vi "RPNSolver.vi"(7 "error in":errorcluster, 9 "Variable Value Array":sgl[](array[numeric]), 10 "Parsed Expression In":T1) -> (0 "error out":errorcluster, 2 "Numeric":sgl format="%#_18f", 3 "Parsed Expression Out":T1)   [LabVIEW 2014, in "MathLoop.lvlib"]
doc: "Resuelve las operaciones matemáticas."
uses:
  MathLoop.lvlib
  TypeDefs/ParsedExpression.ctl
  TypeDefs/typeMed.ctl
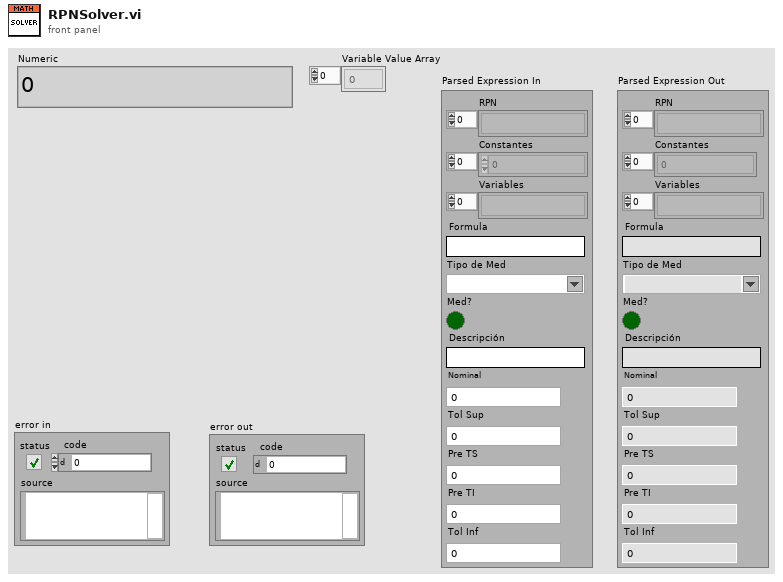
[diagram p1: front panel]
types:
  T1 = typedef "MathLoop.lvlib/ParsedExpression.ctl" = cluster{"RPN ":string[], "Constantes":sgl[], "Variables":string[], "Formula":string, "Tipo de Med":T2, "Med?":bool, "Descripción":string, "Nominal":sgl, "Tol Sup":sgl, "Pre TS":sgl, "Pre TI":sgl, "Tol Inf":sgl}
  T2 = typedef "MathLoop.lvlib/typeMed.ctl" = string
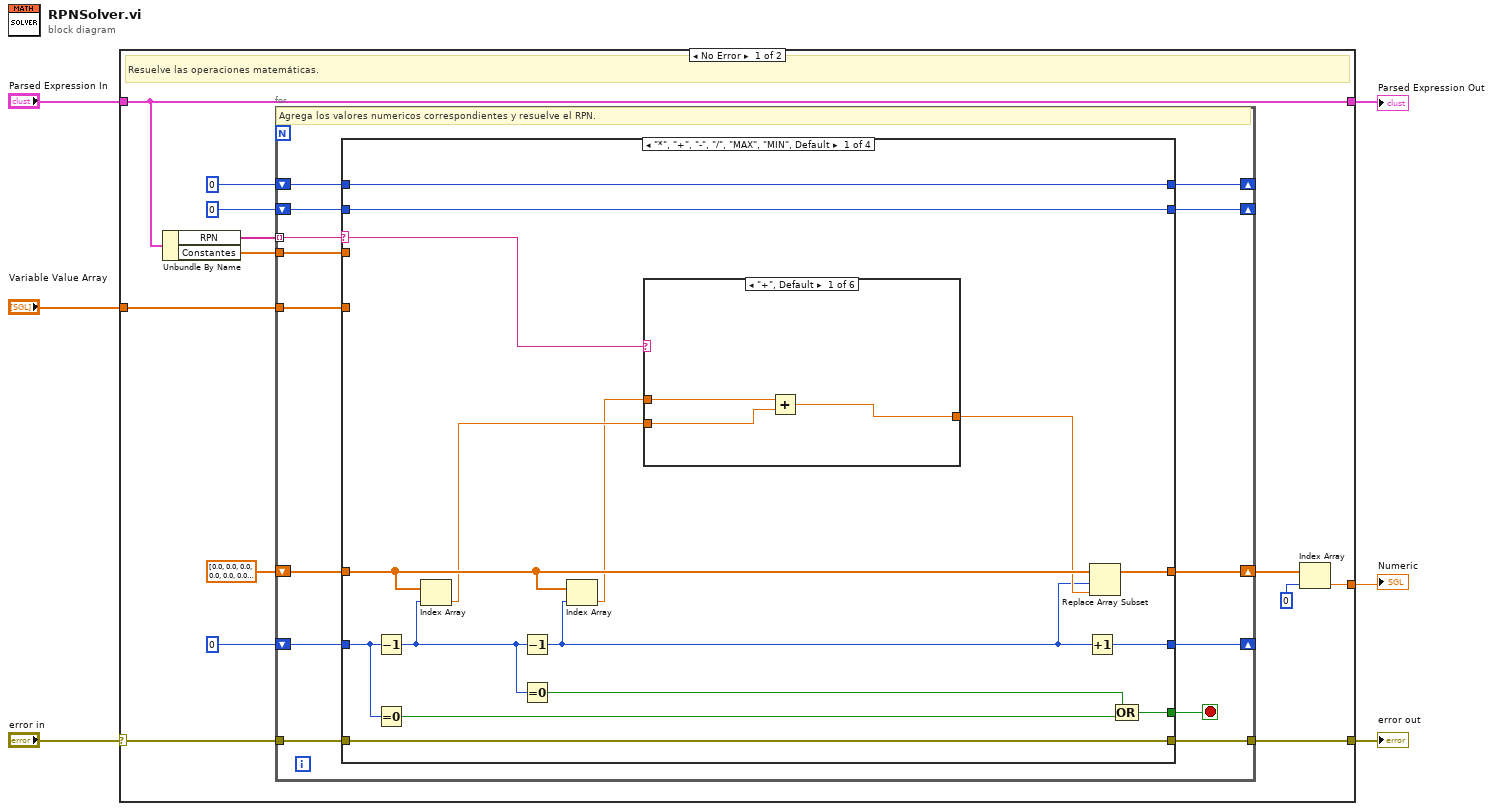
[diagram p0: block diagram]
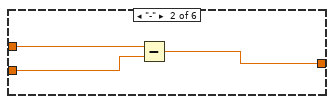
[diagram p2: hidden frame]
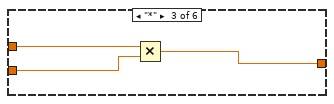
[diagram p3: hidden frame]
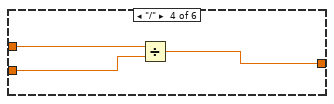
[diagram p4: hidden frame]
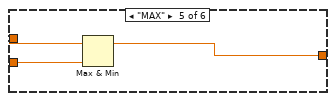
[diagram p5: hidden frame]
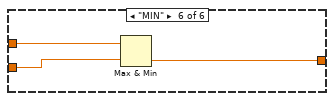
[diagram p6: hidden frame]
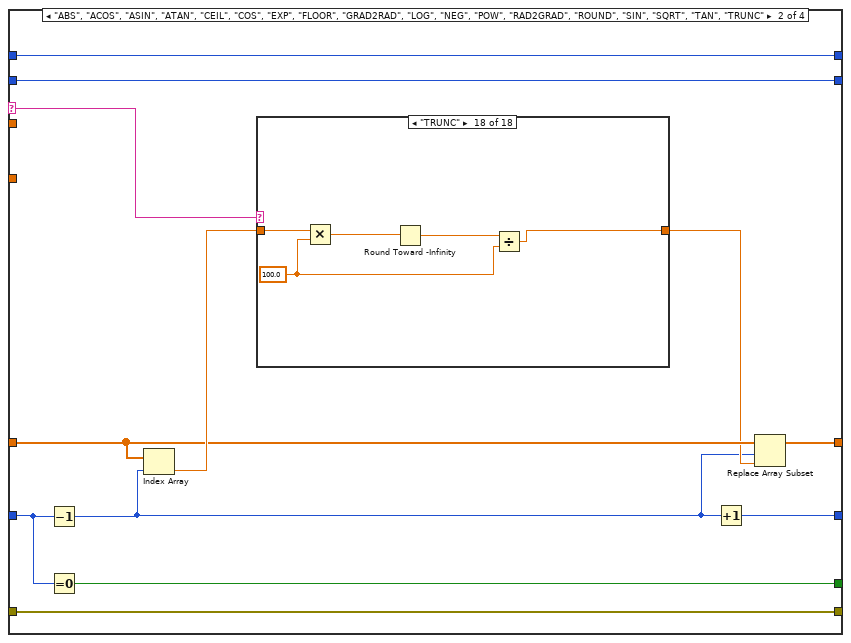
[diagram p7: hidden frame]
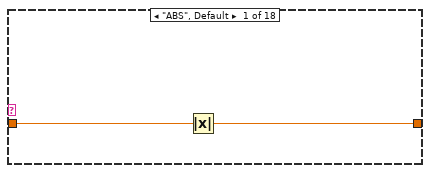
[diagram p8: hidden frame]
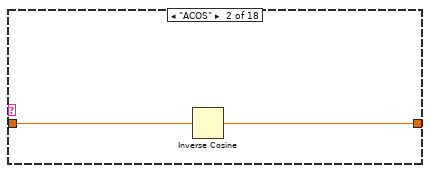
[diagram p9: hidden frame]
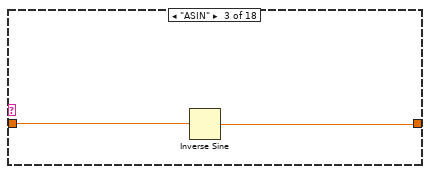
[diagram p10: hidden frame]
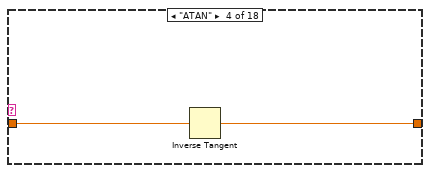
[diagram p11: hidden frame]
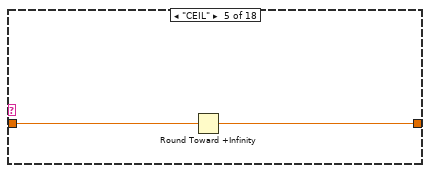
[diagram p12: hidden frame]
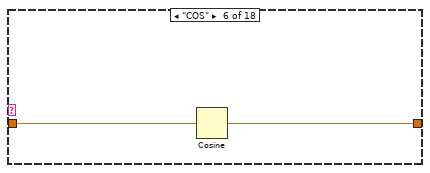
[diagram p13: hidden frame]
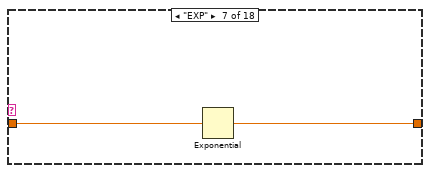
[diagram p14: hidden frame]
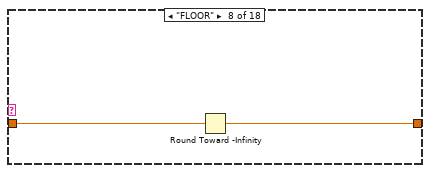
[diagram p15: hidden frame]
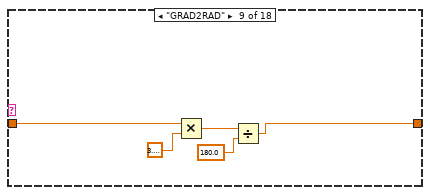
[diagram p16: hidden frame]
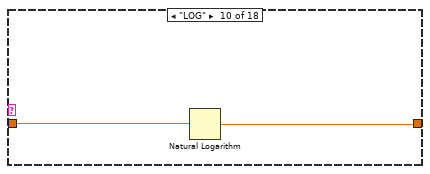
[diagram p17: hidden frame]
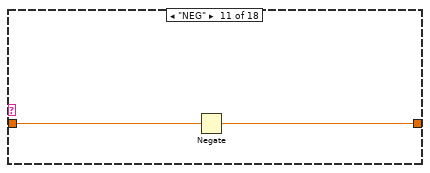
[diagram p18: hidden frame]
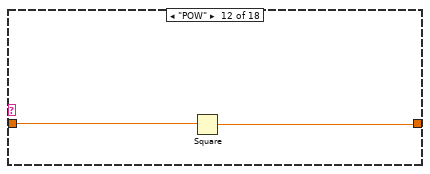
[diagram p19: hidden frame]
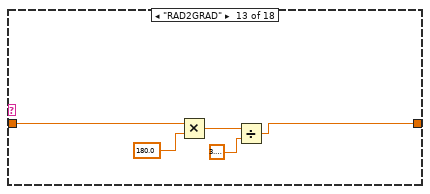
[diagram p20: hidden frame]
diagram:
  n1 = case shown="No Error" "error in" {
    selector: "error in" -> [w8 w147]
    tunnel: [w7 w147] -> w6
    tunnel: "Parsed Expression In" -> [w17 w146]
    tunnel: [w17 w146] -> w2
    tunnel: [w13 sgl 0.0] -> w4
    tunnel: "Variable Value Array" -> [w12 _]
    frame No Error {
      # "Resuelve las operaciones matemáticas."
      n2 = Unbundle By Name(w17) -> ("RPN"=w18:string[], "Constantes"=w16:sgl[])
      n3 = for {
        tunnel: w16 -> [w31]
        tunnel: w18 -> [w32] mode=indexing
        shift-right: [w29] -> _
        shift-left: 0 -> [w30]
        tunnel: w12 -> [w28]
        shift-right: [w27] -> _
        shift-left: 0 -> [w26]
        shift-right: [w25] -> w10
        shift-left: sgl[] [0.0, 0.0, 0.0, 0.0, 0.0, 0.0, 0.0, 0.0, 0.0, 0.0, 0.0, 0.0, 0.0, 0.0, 0.0, 0.0] -> [w24]
        shift-right: [w22] -> _
        shift-left: u8 0 -> [w23]
        tunnel: w8 -> [w21]
        tunnel: [w20] -> w7
        stop <- w33 stop-if-true
        # "Agrega los valores numericos correspondientes y resuelve el RPN."
        n4 = case shown="\"*\", \"+\", \"-\", \"/\", \"MAX\", \"MIN\", Default" w32 {
          selector: w32 -> [w49 w79 _ _]
          tunnel: [w48 w74 _ _] -> w33
          tunnel: w31 -> [_ _ w134 _]
          tunnel: w30 -> [w47 w78 w132 w142]
          tunnel: [w47 w78 w133 w142] -> w29
          tunnel: w28 -> [_ _ _ w144]
          tunnel: w26 -> [w46 w77 w131 w135]
          tunnel: [w46 w77 w131 w143] -> w27
          tunnel: w24 -> [w43 w73 w130 w140]
          tunnel: [w42 w71 w129 w138] -> w25
          tunnel: w23 -> [w45 w75 w126 w137]
          tunnel: [w35 w70 w127 w141] -> w22
          tunnel: w21 -> [w34 w68 w125 w136]
          tunnel: [w34 w68 w125 w136] -> w20
          frame "*", "+", "-", "/", "MAX", "MIN", Default {
            n5 = Decrement(x=w45) -> (x-1=w44:u8)
            n6 = Equal To 0?(x=w45) -> (x = 0?=w38:bool)
            n7 = Index Array(array=w43, index=w44) -> (element=w40:sgl)
            n8 = Decrement(x=w44) -> (x-1=w36:u8)
            n9 = Equal To 0?(x=w44) -> (x = 0?=w37:bool)
            n10 = Index Array(array=w43, index=w36) -> (element=w39:sgl)
            n11 = case shown="\"+\", Default" w49 {
              tunnel: w40 -> [w51 w54 w57 w60 w63 w66]
              tunnel: w39 -> [w52 w55 w58 w61 w64 w67]
              tunnel: [w50 w53 w56 w59 w62 w65] -> w41
              frame "+", Default {
                n12 = Add(x=w52, y=w51) -> (x+y=w50:sgl)
              }
              frame "-" {
                n13 = Subtract(x=w55, y=w54) -> (x-y=w53:sgl)
              }
              frame "*" {
                n14 = Multiply(x=w58, y=w57) -> (x*y=w56:sgl)
              }
              frame "/" {
                n15 = Divide(x=w61, y=w60) -> (x/y=w59:sgl)
              }
              frame "MAX" {
                n16 = Max & Min(x=w64, y=w63) -> (max(x,y)=w62:sgl)  [unwired: 1 out]
              }
              frame "MIN" {
                n17 = Max & Min(x=w67, y=w66) -> (min(x,y)=w65:sgl)  [unwired: 1 out]
              }
            }
            n18 = Increment(x=w36) -> (x+1=w35:u8)
            n19 = Replace Array Subset(array=w43, new element=w41, index=w36) -> (w42:sgl[])
            n20 = Compound Arithmetic op=OR(w37, w38) -> (w48:bool)
          }
          frame "ABS", "ACOS", "ASIN", "ATAN", "CEIL", "COS", "EXP", "FLOOR", "GRAD2RAD", "LOG", "NEG", "POW", "RAD2GRAD", "ROUND", "SIN", "SQRT", "TAN", "TRUNC" {
            n21 = Decrement(x=w75) -> (x-1=w69:u8)
            n22 = Equal To 0?(x=w75) -> (x = 0?=w74:bool)
            n23 = Index Array(array=w73, index=w69) -> (element=w76:sgl)
            n24 = case shown="\"TRUNC\"" w79 {
              tunnel: w76 -> [w81 w83 w85 w87 w89 w91 w93 w95 w97 w102 w104 w106 w111 w113 w115 w117 w119 w124]
              tunnel: [w80 w82 w84 w86 w88 w90 w92 w94 w96 w101 w103 w105 w107 w112 w114 w116 w118 w120] -> w72
              frame "ABS", Default {
                n25 = Absolute Value(x=w81) -> (abs(x)=w80:sgl)
              }
              frame "ACOS" {
                n26 = Inverse Cosine(1:w83) -> (0:w82:sgl)
              }
              frame "ASIN" {
                n27 = Inverse Sine(1:w85) -> (0:w84:sgl)
              }
              frame "ATAN" {
                n28 = Inverse Tangent(1:w87) -> (0:w86:sgl)
              }
              frame "CEIL" {
                n29 = Round Toward +Infinity(x=w89) -> (ceil(x): smallest int >= x=w88:sgl)
              }
              frame "COS" {
                n30 = Cosine(x=w91) -> (cos(x)=w90:sgl)
              }
              frame "EXP" {
                n31 = Exponential(1:w93) -> (0:w92:sgl)
              }
              frame "FLOOR" {
                n32 = Round Toward -Infinity(1:w95) -> (0:w94:sgl)
              }
              frame "GRAD2RAD" {
                n33 = Multiply(x=w97, y=sgl 3.1415927) -> (x*y=w100:sgl)
                n34 = Divide(x=w100, y=sgl 180.0) -> (x/y=w96:sgl)
              }
              frame "LOG" {
                n35 = Natural Logarithm(1:w102) -> (0:w101:sgl)
              }
              frame "NEG" {
                n36 = Negate(x=w104) -> (-x=w103:sgl)
              }
              frame "POW" {
                n37 = Square(x=w106) -> (x^2=w105:sgl)
              }
              frame "RAD2GRAD" {
                n38 = Multiply(x=w111, y=sgl 180.0) -> (x*y=w110:sgl)
                n39 = Divide(x=w110, y=sgl 3.1415927) -> (x/y=w107:sgl)
              }
              frame "ROUND" {
                n40 = Round To Nearest(number=w113) -> (nearest integer value=w112:sgl)
              }
              frame "SIN" {
                n41 = Sine(x=w115) -> (sin(x)=w114:sgl)
              }
              frame "SQRT" {
                n42 = Square Root(x=w117) -> (sqrt(x)=w116:sgl)
              }
              frame "TAN" {
                n43 = Tangent(1:w119) -> (0:w118:sgl)
              }
              frame "TRUNC" {
                w121 = sgl 100.0 ("y")
                n44 = Multiply(x=w124, y=w121) -> (x*y=w123:sgl)
                n45 = Round Toward -Infinity(1:w123) -> (0:w122:sgl)
                n46 = Divide(x=w122, y=w121) -> (x/y=w120:sgl)
              }
            }
            n47 = Increment(x=w69) -> (x+1=w70:u8)
            n48 = Replace Array Subset(array=w73, new element=w72, index=w69) -> (w71:sgl[])
          }
          frame "Constante" {
            n49 = Index Array(array=w134, index=w132) -> (element=w128:sgl)
            n50 = Replace Array Subset(array=w130, new element=w128, index=w126) -> (w129:sgl[])
            n51 = Increment(x=w126) -> (x+1=w127:u8)
            n52 = Increment(x=w132) -> (x+1=w133:i32)
          }
          frame "Variable" {
            n53 = Index Array(array=w144, index=w135) -> (element=w139:sgl)
            n54 = Replace Array Subset(array=w140, new element=w139, index=w137) -> (w138:sgl[])
            n55 = Increment(x=w137) -> (x+1=w141:u8)
            n56 = Increment(x=w135) -> (x+1=w143:i32)
          }
        }
      }
      n57 = Index Array(array=w10, index=0) -> (element=w13:sgl)
    }
    frame Error {
    }
  }
  "error out" <- w6
  "Numeric" <- w4
  "Parsed Expression Out" <- w2
